vi "Inspect Tell.vi"(4 "Unified Actor Alias":string, 9 "Teller":T1 {"Absolute Time" format="%<%x %.3X>T"}, 10 "Msg":refnum<class "Msg.lvclass">, 11 "Actor in":refnum<class "Actor.lvclass">) -> (3 "Actor out":refnum<class "Actor.lvclass">)   [LabVIEW 2020, in "jettl.lvlib" / "Actor.lvclass"]
uses:
  Actor.lvclass
  Unified Actor Relation.ctl
  jettl.lvlib
  Teller.ctl
  Msg/Msg.lvclass
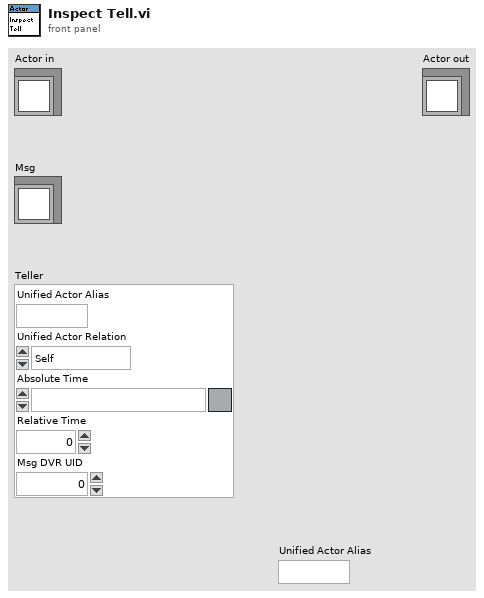
[diagram p1: front panel]
types:
  T1 = typedef "jettl.lvlib/Teller.ctl" = cluster{"Unified Actor Alias":string, "Unified Actor Relation":T2, "Absolute Time":timestamp, "Relative Time":dbl, "Msg DVR UID":i32}
  T2 = typedef "jettl.lvlib/Unified Actor Relation.ctl" = enum16{"Self", "Parent", "Child"}
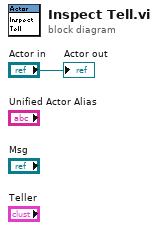
[diagram p0: block diagram]
diagram:
  "Actor out" <- "Actor in"
